vi "Deadband.vi"(10 "Cluster":T1={"Drive Forward Input "=0.0, "Drive Twist Input"=0.0, "Drive Output"=0.0, "Drivetwist Output"=0.0, "Left Joystick Buttons"=[FALSE, FALSE, FALSE, FALSE, FALSE, FALSE, FALSE, FALSE, FALSE, FALSE, FALSE, FALSE], "Left Joystick Axis"=[-0.007874015748031496, -0.0, -0.0, 0.18110236220472442], "Right Joystick Axis"=[], "Right Joystick Button"=[], "Arm Encoder"=4.0, "Left Drive Encoder"=0.0, "Right Drive Encoder"=1337462.0, "Gyro Angle "=188.0419921875, "Arm Joystick Output  "=0.0, "Line Follower L, C, R "=[TRUE, TRUE, TRUE], "Line follow?"=FALSE, " Climb Solenoid"=FALSE, "Wrist Encoder Count"=0.0, "Wrist Joystick Output"=0.0, "Ball Encoder Count"=0.0, "Ball Output"=0.0, "Climb Encoder"=0.0, "Climb Motor Output"=0.0, " Hatch Solenoid"=FALSE, "Arm Setpoint "=0.0, "Wrist Setpoint "=0.0, "Arm Joystick Enabled?"=FALSE, "Wrist Joystick Enabled"=FALSE, "Vision String"="", "Left Joystick POVs"=[-1]}, 11 "Twiest Input":dbl=-0.0) -> (2 "Dead Band Zone":bool=TRUE, 3 "Tweest Interpreted":dbl)   [LabVIEW 2018]
uses:
  TypeDefs/Teleop Data Cluster.ctl
  TypeDefs/Joystick Buttons.ctl
panel:
  in  "normal mult":dbl=0.4 format="%#_13g"
  in  "cube multiplier":dbl=0.55 format="%#_13g"
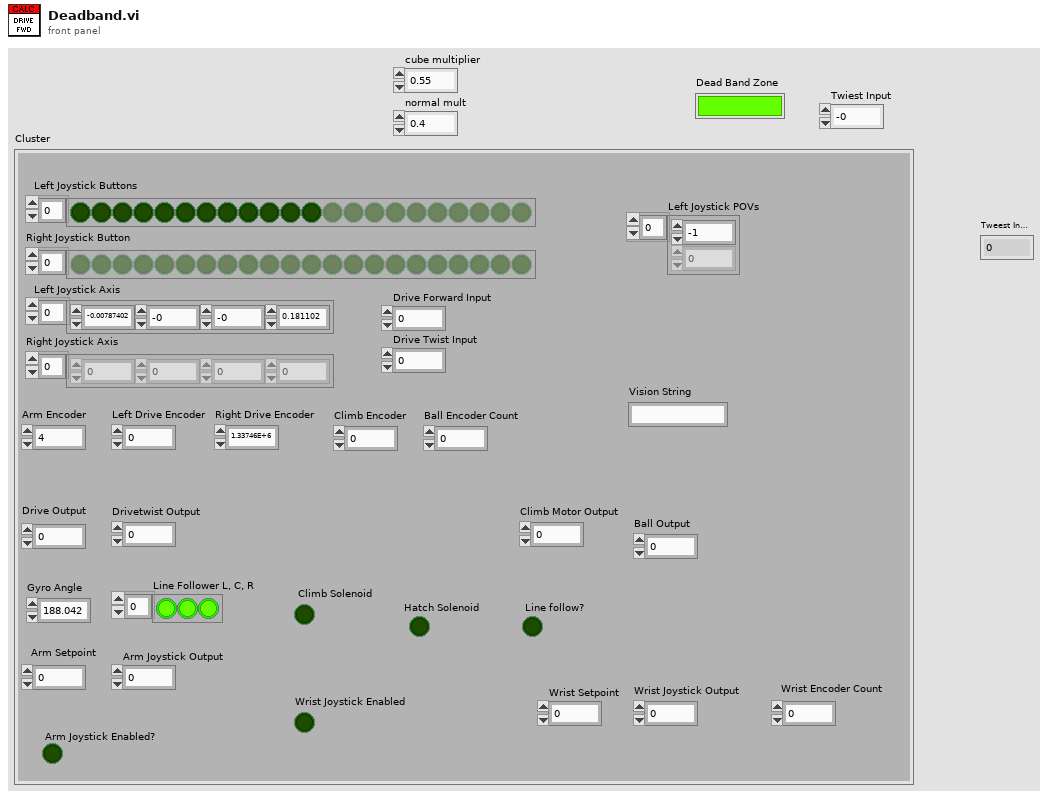
[diagram p1: front panel]
types:
  T1 = typedef "Teleop Data Cluster.ctl" = cluster{"Drive Forward Input ":dbl, "Drive Twist Input":dbl, "Drive Output":dbl, "Drivetwist Output":dbl, "Left Joystick Buttons":bool[], "Left Joystick Axis":dbl[], "Right Joystick Axis":dbl[], "Right Joystick Button":bool[], "Arm Encoder":dbl, "Left Drive Encoder":dbl, "Right Drive Encoder":dbl, "Gyro Angle ":dbl, "Arm Joystick Output  ":dbl, "Line Follower L, C, R ":bool[], "Line follow?":bool, " Climb Solenoid":bool, "Wrist Encoder Count":dbl, "Wrist Joystick Output":dbl, "Ball Encoder Count":dbl, "Ball Output":dbl, "Climb Encoder":dbl, "Climb Motor Output":dbl, " Hatch Solenoid":bool, "Arm Setpoint ":dbl, "Wrist Setpoint ":dbl, "Arm Joystick Enabled?":bool, "Wrist Joystick Enabled":bool, "Vision String":string, "Left Joystick POVs":i16[]}
  T2 = typedef "Joystick Buttons.ctl" = enum16{"Trigger", "Thumb", "Top 3", "Top 4", "Top 5", "Top 6", "Bottom 7", "Bottom 8", "Bottom 9", "Bottom 10", "Bottom 11", "Bottom 12"}
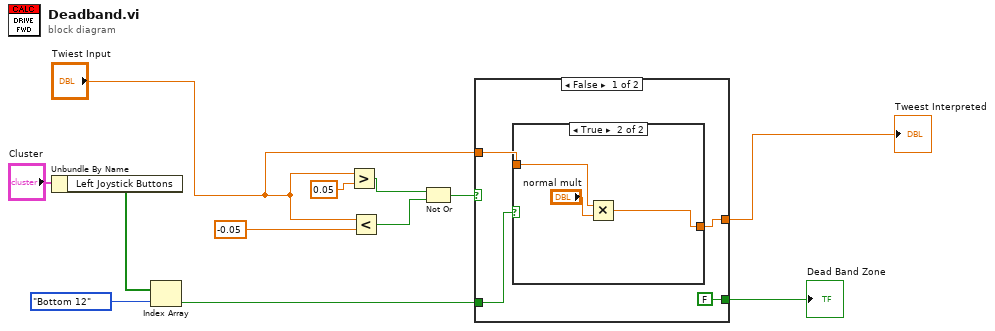
[diagram p0: block diagram]
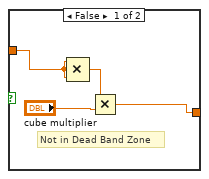
[diagram p2: hidden frame]
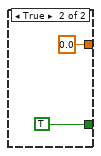
[diagram p3: hidden frame]
diagram:
  n1 = Unbundle By Name("Cluster") -> ("Left Joystick Buttons"=w2:bool[])
  n2 = Index Array(array=w2, index=Joystick_Buttons."Bottom 12" ("Enum")) -> (element=w1:bool)
  n3 = Greater?(x="Twiest Input", y=0.05) -> (0:w10:bool)
  n4 = Less?(x="Twiest Input", y=-0.05) -> (x < y?=w9:bool)
  n5 = Not Or(1:w9, 2:w10) -> (0:w8:bool)
  n6 = case shown="False" w8 {
    tunnel: [FALSE TRUE] -> w7
    tunnel: [w13 0.0 ("Drive Forward Input")] -> w5
    tunnel: "Twiest Input" -> [w15 _]
    tunnel: w1 -> [w14 _]
    frame False {
      n7 = case shown="True" w14 {
        tunnel: w15 -> [w18 w22]
        tunnel: [w17 w21] -> w13
        frame False {
          # "Not in Dead Band Zone"
          n8 = Compound Arithmetic op=MULTIPLY(w18, w18, w18) -> (w19:dbl)
          n9 = Multiply(x=w19, y="cube multiplier") -> (x*y=w17:dbl)
        }
        frame True {
          n10 = Multiply(x=w22, y="normal mult") -> (x*y=w21:dbl)
        }
      }
    }
    frame True {
    }
  }
  "Dead Band Zone" <- w7
  "Tweest Interpreted" <- w5
